vi "Open.vi"(8 "error in":errorcluster, 10 "Baudrate":u32=500000, 11 "CanHandleIn":T1) -> (0 "error out":errorcluster, 3 "CanHandleOut":T1)   [LabVIEW 2011, in "Konvolucio MCAN120803.lvlib"]
doc: "Opens a new CAN bus connection with specified baudrate."
uses:
  <instrlib>/Konvolucio MCAN120803/Konvolucio MCAN120803.lvlib
  <instrlib>/Konvolucio MCAN120803/Types/CanHandleType.ctl
  C:/Program Files/National Instruments/LabVIEW 2011/instr.lib/Konvolucio MCAN120803/Private/Konvolucio.MCAN120803.API.dll
  Private/Konvolucio.MCAN120803.API.dll
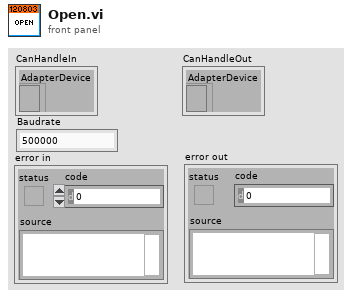
[diagram p1: front panel]
types:
  T1 = typedef "Konvolucio MCAN120803.lvlib/CanHandleType.ctl" = cluster{"AdapterDevice":refnum<k24>}
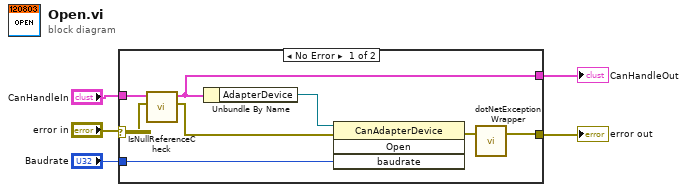
[diagram p0: block diagram]
diagram:
  n1 = case shown="No Error" "error in" {
    selector: "error in" -> [w6 w15]
    tunnel: "Baudrate" -> [w13 _]
    tunnel: [w11 w15] -> w4
    tunnel: "CanHandleIn" -> [w8 w14]
    tunnel: [w9 w14] -> w1
    frame No Error {
      n2 = call <instrlib>:"IsNullReferenceCheck.vi"("error in"=w6, "MCanHandleIn"=w8) -> ("error out"=w7:errorcluster, "MCanHandleOut"=w9:T1)  [unwired: 5 in]
      n3 = Unbundle By Name(w9) -> ("AdapterDevice"=w12:refnum<k24>)
      n4 = invoke class="CanAdapterDevice" method="Open"(reference=w12, error in=w7, "baudrate"=w13) -> (error out=w10:errorcluster)  [unwired: 1 in, 3 out]
      n5 = call <instrlib>:"dotNetExceptionWrapper.vi"("error in"=w10) -> ("error out"=w11:errorcluster)  [unwired: 2 in]
    }
    frame Error {
    }
  }
  "error out" <- w4
  "CanHandleOut" <- w1
